vi "Emballage_BDD_produit_ART_BDD.vi"(8 "Error in":errorcluster caption="Error in (no error)", 11 "ID_ARTICLE":i32) -> (0 "Error out":errorcluster, 3 "ART produit":string)   [LabVIEW 2020]
uses:
  Modules/FS/60_FS_Controles/60_FS_SetGet.ctl
  <vilib>/addons/database/Connection.llb/DB Tools Open Connec (Path).vi
  <vilib>/addons/database/Connection.llb/Conn Execute.vi
  <vilib>/addons/database/Recordset.llb/Rec Fetch Recordset Data (R).vi
  <vilib>/addons/database/Recordset.llb/Rec Destroy - Connection.vi
  <vilib>/addons/database/NI_Database_API.lvlib
panel:
  out "données":string[][](array[string])
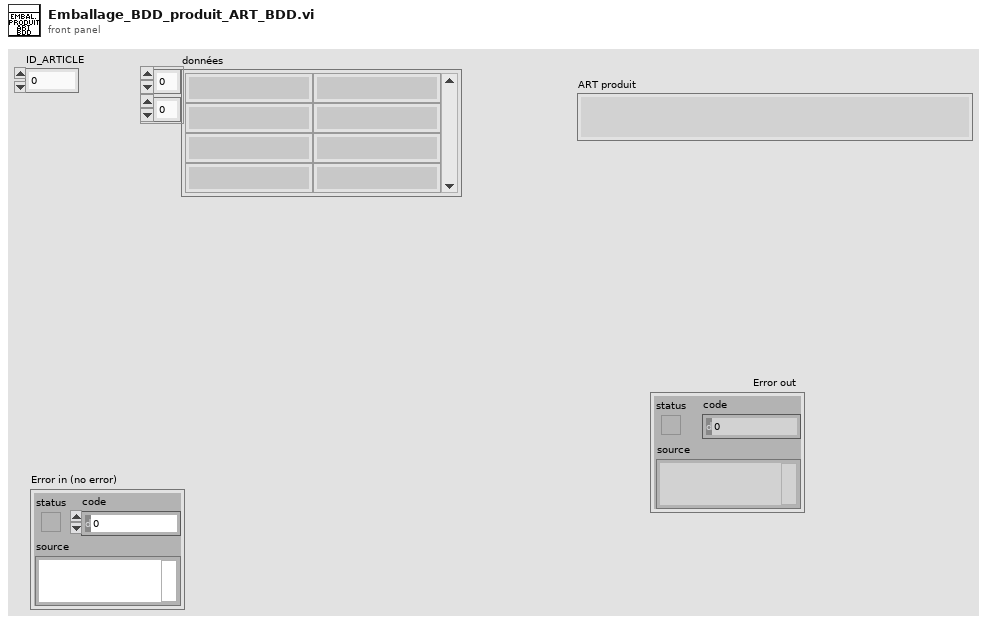
[diagram p1: front panel]
types:
  T1 = typedef "60_FS_SetGet.ctl" = enum16{"set", "get"}
  T2 = typedef "60_FS_CLT_Chemins.ctl" = cluster{"Racine_local":path, "Racine_reseau":path, "Racine_Support_Application":path, "Fichier_Journalisation":path, "Connexion_BDD_VSX":path, "Connexion_BDD_PLZ":path}
  T3 = typedef "NI_Database_API.lvlib/Conn ObjectReference.ctl" = refnum<k1>
  T4 = typedef "NI_Database_API.lvlib/Rec ObjectReference.ctl" = refnum<k1>
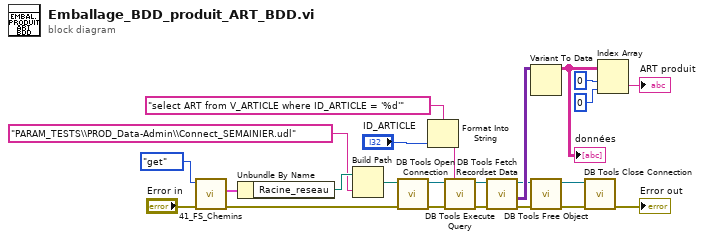
[diagram p0: block diagram]
diagram:
  n1 = call "41_FS_Chemins.vi"("error in (no error)"="Error in", "SetGet"=60_FS_SetGet."get") -> ("error out"=w24:errorcluster, "CLT_Chemins_out"=w21:T2)  [unwired: 8 in]
  n2 = Unbundle By Name(w21) -> ("Racine_reseau"=w23:path)
  n3 = Build Path(base path=w23, name or relative path="PARAM_TESTS\\PROD_Data-Admin\\Connect_SEMAINIER.udl" ("nom ou chemin relatif")) -> (appended path=w4:path)
  n4 = call-poly <vilib>:"DB Tools Open Connection.vi"("error in (no error)"=w24, "connection information"=w4) -> ("error out"=w9:errorcluster, "connection reference"=w8:T3)  [unwired: 6 in]
  n5 = Format Into String(format string="select ART from V_ARTICLE where ID_ARTICLE = '%d'" ("SQL query"), "ID_ARTICLE") -> (resulting string=w2:string)  [unwired: 2 in, 1 out]
  n6 = call-poly <vilib>:"DB Tools Execute Query.vi"("error in (no error)"=w9, "SQL query"=w2, "connection reference"=w8) -> ("error out"=w12:errorcluster, "recordset reference"=w14:T4)  [unwired: 5 in]
  n7 = call-poly <vilib>:"DB Tools Fetch Recordset Data.vi"("error in (no error)"=w12, "recordset reference"=w14) -> ("error out"=w13:errorcluster, "recordset data"=w16:variant[][], "recordset reference out"=w15:T4)  [unwired: 3 in]
  n8 = Variant To Data(Variant=w16) -> (data=w17:string[][])  [unwired: 2 in, 1 out]
  "données" <- w17
  n9 = call-poly <vilib>:"DB Tools Free Object.vi"("error in (no error)"=w13, "recordset reference"=w15) -> ("error out"=w10:errorcluster, "connection reference"=w11:T3)  [unwired: 8 in]
  n10 = call <vilib>:"DB Tools Close Connection.vi"("error in (no error)"=w10, "connection reference"=w11) -> ("error out"=→"Error out":errorcluster)  [unwired: 5 in]
  n11 = Index Array(array=w17, index (row)=0 ("indice (ligne)"), index (col)=0 ("indice désactivé (col)")) -> (element=→"ART produit":string)
